vi "Number to Proper English text - 0 to 1000.vi"(8 "error in (no error)":errorcluster, 11 "Positive integer <= 1000":u16) -> (0 "error out":errorcluster, 3 "Integer written in English":string)   [LabVIEW 2021, in "Project Euler.lvlib"]
uses:
  Project Euler.lvlib
panel:
  # "Development\ncontrols/indicators useful for development and testing, but which are not outputs of the VI"
  # "Input\nInputs to the VI"
  # "Output\nOutputs of the VI"
  # "Description\n\nBlank VI with error handling case. \n\nSummarize the use of this VI in this space."
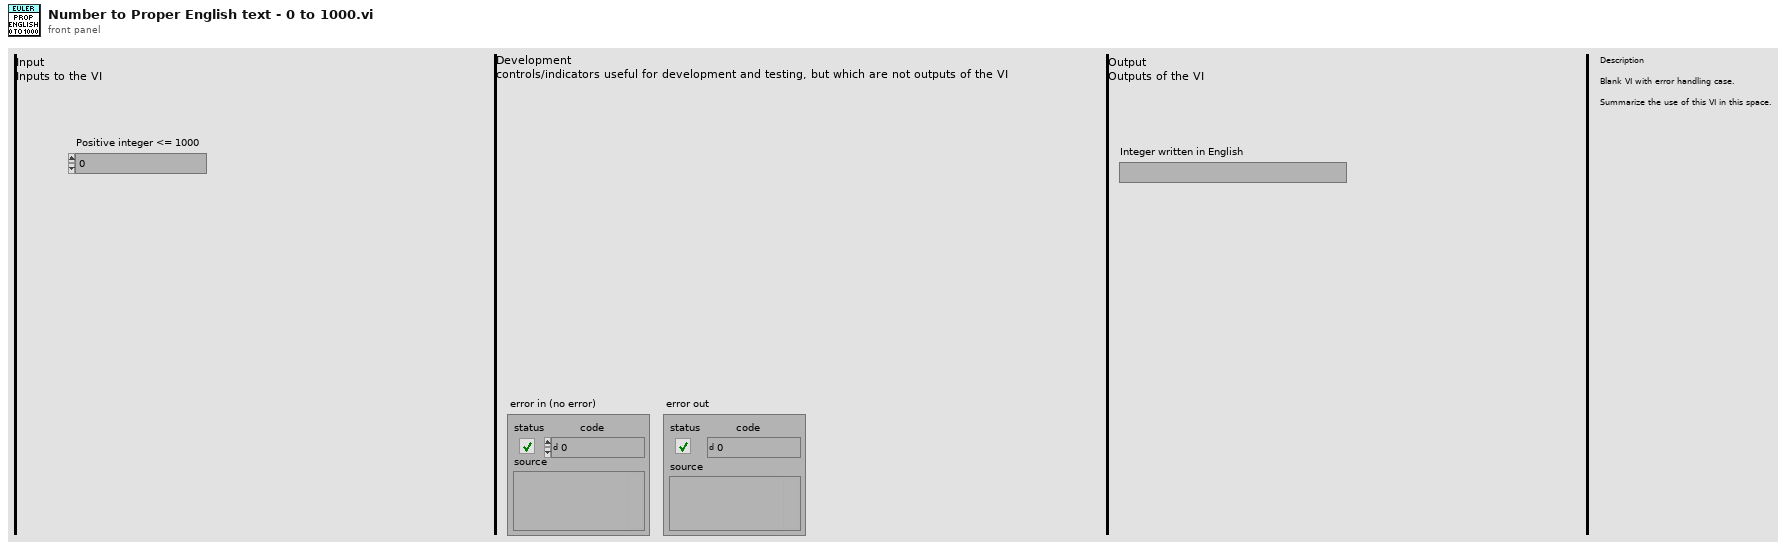
[diagram p1: front panel]
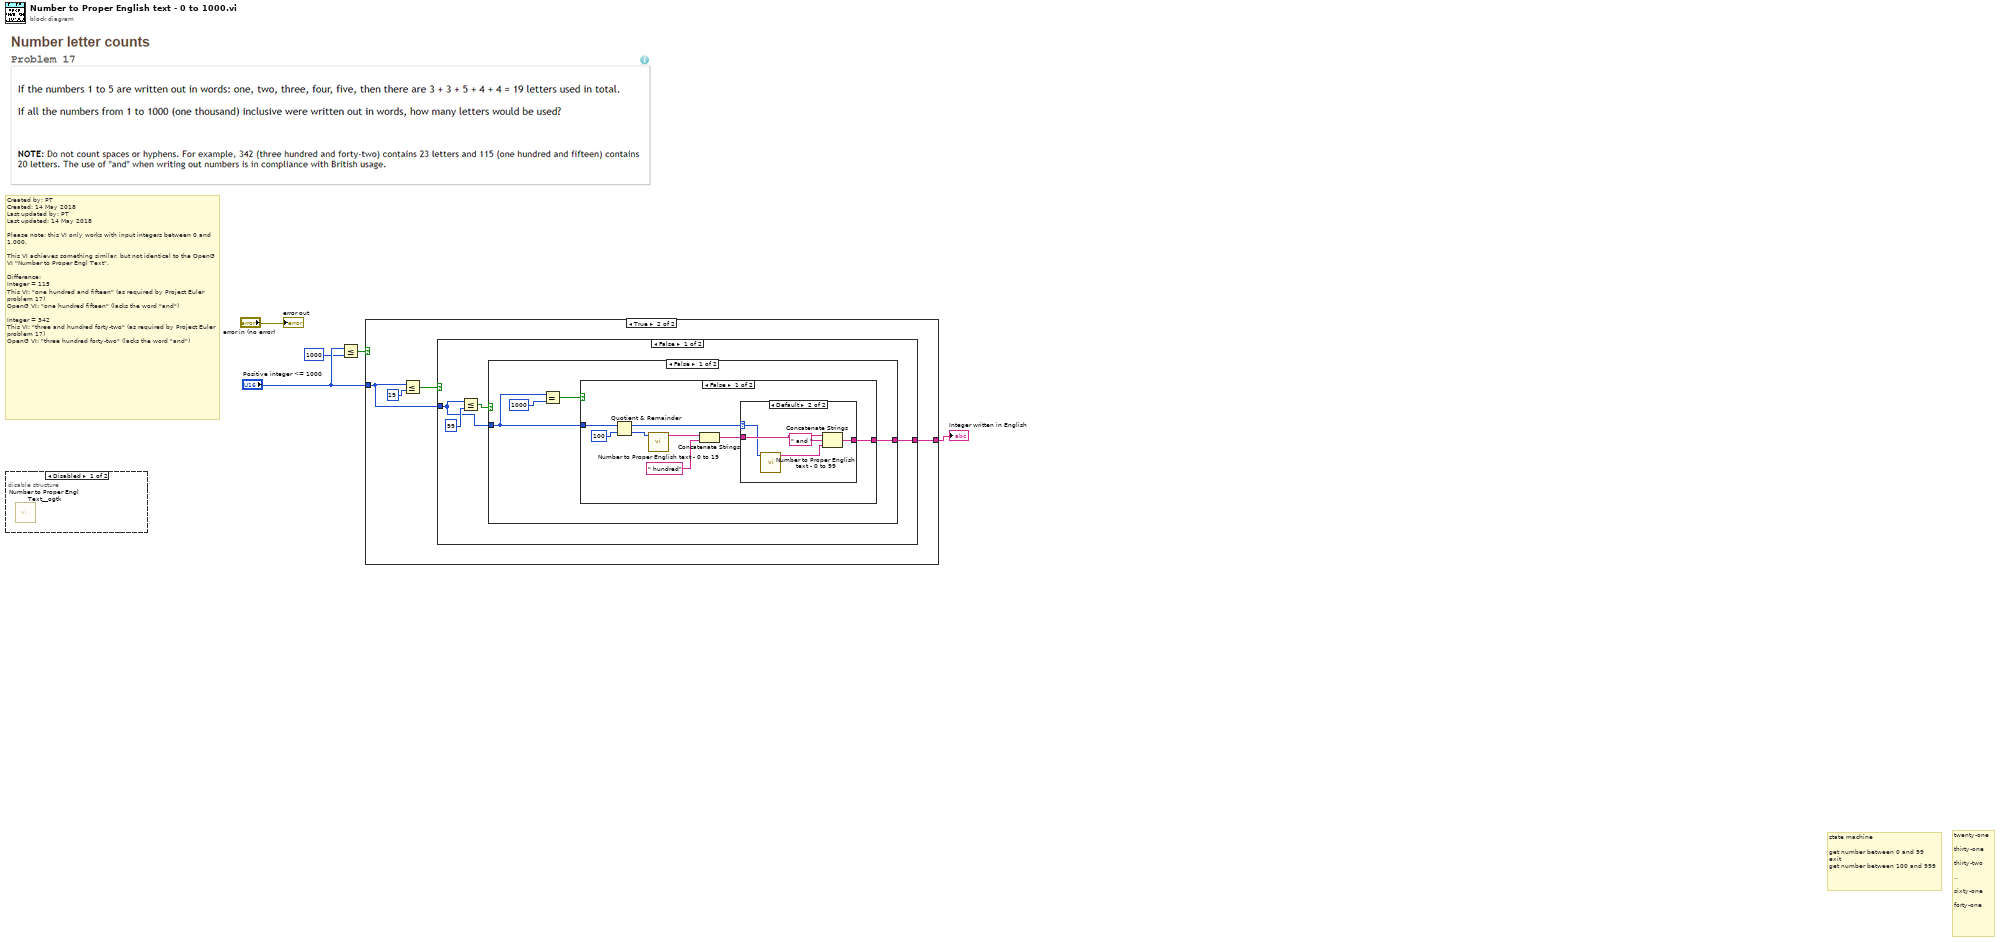
[diagram p0: block diagram]
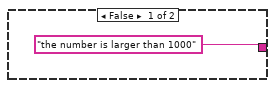
[diagram p2: hidden frame]
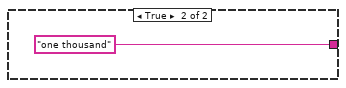
[diagram p4: hidden frame]
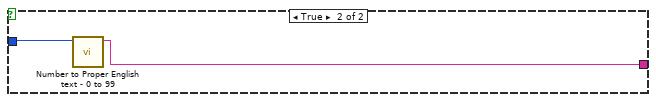
[diagram p5: hidden frame]
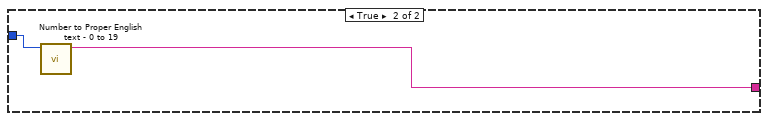
[diagram p6: hidden frame]
diagram:
  # "state machine\n\nget number between 0 and 99\nexit\nget number between 100 and 999"
  # "twenty-one\n\nthirty-one\n\nthirty-two\n\n..\n\nsixty-one\n\nforty-one"
  # "Created by: PT\nCreated: 14 May 2018\nLast updated by: PT\nLast updated: 14 May 2018\n\nPlease note: this VI only works with input integers between 0 and 1,000.\n\nThis VI achieves something similar, but not identical to the OpenG VI \"Number to Proper Engl Text\".\n\nDifference:\nInteger = 115\nThis VI: \"one hundred and fifteen\" (as required by Project Euler problem 17)\nOpenG VI: \"one hundred fifteen\" (lacks the word \"and\")\n\nInteger = 342\nThis VI: \"three and hundred forty-two\" (as required by Project Euler problem 17)\nOpenG VI: \"three hundred forty-two\" (lacks the word \"and\")"
  n1 = disable-structure shown="Disabled" {
    frame Disabled {
      n2 = call <userlib>:"Number to Proper Engl Text__ogtk.vi"() -> ()  [unwired: 5 in, 1 out]
    }
    frame Enabled {
    }
  }
  n3 = Less Or Equal?(x="Positive integer <= 1000", y=u16 1000) -> (x <= y?=w1:bool)
  n4 = case shown="True" w1 {
    tunnel: ["the number is larger than 1000" w7] -> w4
    tunnel: "Positive integer <= 1000" -> [_ w8]
    frame False {
    }
    frame True {
      n5 = Less Or Equal?(x=w8, y=u16 19) -> (x <= y?=w9:bool)
      n6 = case shown="False" w9 {
        tunnel: w8 -> [w11 w37]
        tunnel: [w12 w36] -> w7
        frame False {
          n7 = Less Or Equal?(x=w11, y=u16 99) -> (x <= y?=w13:bool)
          n8 = case shown="False" w13 {
            tunnel: [w18 w35] -> w12
            tunnel: w11 -> [w17 w34]
            frame False {
              n9 = Equal?(x=w17, y=u16 1000) -> (x = y?=w15:bool)
              n10 = case shown="False" w15 {
                tunnel: w17 -> [w26 _]
                tunnel: [w19 "one thousand"] -> w18
                frame False {
                  n11 = Quotient & Remainder(x=w26, y=u16 100) -> (x-y*floor(x/y)=w21:u16, floor(x/y)=w24:u16)
                  n12 = call "Number to Proper English text - 0 to 19.vi"("Positive integer <= 19"=w24) -> ("Integer written in English"=w23:string)  [unwired: 9 in, 1 out]
                  n13 = Concatenate Strings(w23, " hundred" ("string")) -> (w20:string)
                  n14 = case shown="Default" w21 {
                    selector: w21 -> [_ w28]
                    tunnel: w20 -> [w27 w32]
                    tunnel: [w27 w29] -> w19
                    frame 0 {
                    }
                    frame Default {
                      n15 = call "Number to Proper English text - 0 to 99.vi"("Positive integer <= 99"=w28) -> ("Integer written in English"=w30:string)  [unwired: 9 in, 1 out]
                      n16 = Concatenate Strings(w32, " and " ("string"), w30) -> (w29:string)
                    }
                  }
                }
                frame True {
                }
              }
            }
            frame True {
              n17 = call "Number to Proper English text - 0 to 99.vi"("Positive integer <= 99"=w34) -> ("Integer written in English"=w35:string)  [unwired: 9 in, 1 out]
            }
          }
        }
        frame True {
          n18 = call "Number to Proper English text - 0 to 19.vi"("Positive integer <= 19"=w37) -> ("Integer written in English"=w36:string)  [unwired: 9 in, 1 out]
        }
      }
    }
  }
  "Integer written in English" <- w4
  "error out" <- "error in (no error)"
